vi "StateDiagramGraph_Delete.vi"(0 "reference in":refnum<class "StateDiagramGraph.lvclass">, 5 "error in (no error)":errorcluster) -> (14 "reference out":refnum<class "StateDiagramGraph.lvclass">, 15 "# of objects":i32, 19 "error out":errorcluster)   [LabVIEW 2020, in "StateDiagramGraph.lvclass"]
doc: "Deletes a StateDiagramGraph object created with the StateDiagramGraph new VI and returns the contents of the object.\n\n[GOOP 2.0.15]"
uses:
  <resource>/Framework/Providers/Open_GDS/UML/StateDiagramGraph_class/StateDiagramGraph.lvclass
  <vilib>/addons/_goop3.llb/3GOOPStates.ctl
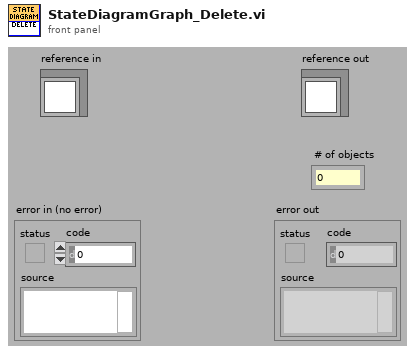
[diagram p1: front panel]
types:
  T1 = typedef "3GOOPStates.ctl" = enum16{"Set", "Get", "New", "Delete", "Clear", "Test and get", "Unlock data", "Information", "Look up existing", "New or look up existing", "Test and get shared", "Get shared", "Set shared", "Unlock shared", "Find dynamic method", "Register dynamic method", "Preload dynamic method", "Probe", "Cast to more generic", "Cast to more specific"}
  T2 = typedef "Graph.lvclass/ObjectReference.ctl" = refnum<k1>
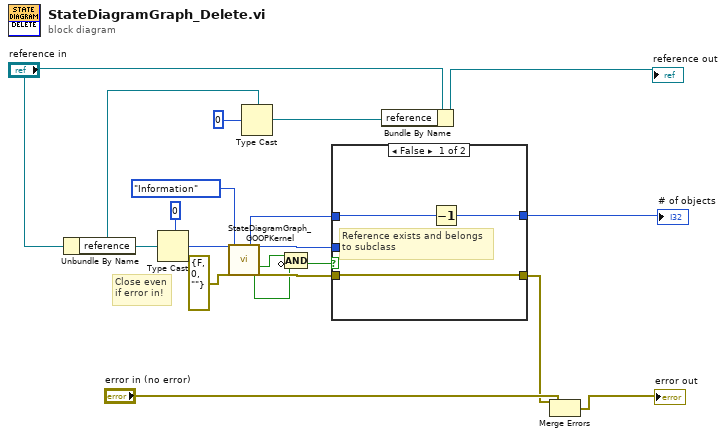
[diagram p0: block diagram]
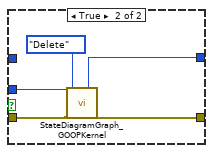
[diagram p2: hidden frame]
diagram:
  # "Close even\nif error in!"
  n1 = Unbundle By Name("reference in") -> ("reference"=w4:T2)
  n2 = Type Cast(type=0, x=w4) -> (*(type *) &x=w15:i32)
  n3 = call <resource>:"StateDiagramGraph_GOOPKernel.vi"("Ref in"=w15, "error in (no error)"=errorcluster {"status"=FALSE, "code"=0, "source"=""}, "Action"=3GOOPStates."Information") -> ("# of objects"=w8:i32, "IsSubclass?"=w12:bool, "Ref out"=w11:i32, "Exists?"=w13:bool, "error out"=w14:errorcluster)  [unwired: 12 in, 8 out]
  n4 = Type Cast(type=w4, x=0) -> (*(type *) &x=w2:T2)
  n5 = Compound Arithmetic op=AND(w13, invert w12) -> (w10:bool)
  n6 = case shown="False" w10 {
    tunnel: [w20 w27] -> w16
    tunnel: [w22 w24] -> w1
    tunnel: w14 -> [w20 w26]
    tunnel: w11 -> [_ w25]
    tunnel: w8 -> [w21 _]
    frame False {
      # "Reference exists and belongs\nto subclass"
      n7 = Decrement(x=w21) -> (x-1=w22:i32)
    }
    frame True {
      n8 = call <resource>:"StateDiagramGraph_GOOPKernel.vi"("Ref in"=w25, "error in (no error)"=w26, "Action"=3GOOPStates."Delete") -> ("# of objects"=w24:i32, "error out"=w27:errorcluster)  [unwired: 12 in, 11 out]
    }
  }
  "# of objects" <- w1
  n9 = Bundle By Name(cluster="reference in", "reference"=w2) -> (→"reference out":refnum<class "StateDiagramGraph.lvclass">)
  n10 = Merge Errors("error in (no error)", w16) -> (→"error out":errorcluster)
